vi "ProcessSpectralBands.vi"(8 "error in (no error)":errorcluster, 11 "tdms ref in":refnum<k34>) -> (0 "error out":errorcluster, 3 "tdms ref out":refnum<k34>)   [LabVIEW 2017, in "DataExplorerSupport.lvlib"]
uses:
  <vilib>/addons/InsightCM/Utilities/DataExplorerSupport/DataExplorerSupport.lvlib
  <vilib>/addons/InsightCM/Utilities/Tdms/Tdms.lvlib
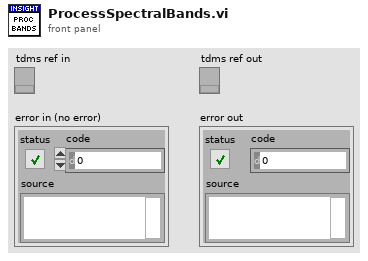
[diagram p1: front panel]
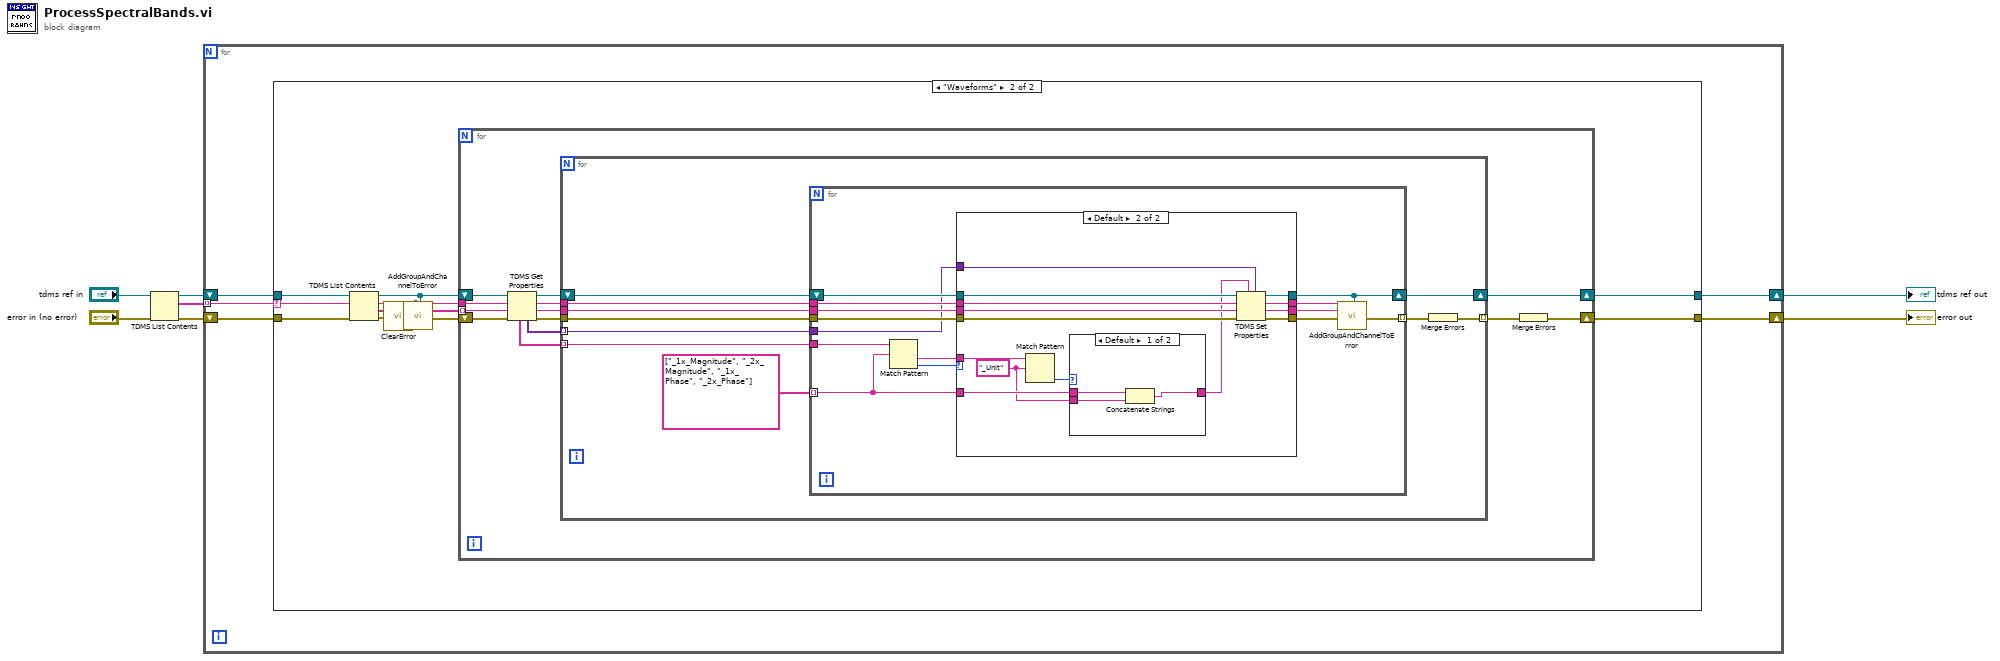
[diagram p0: block diagram]
diagram:
  n1 = TDMS List Contents(4:"error in (no error)", 7:"tdms ref in") -> (0:w2:errorcluster, 2:w1:string[], 3:w4:refnum<k34>)  [unwired: 1 in, 1 out]
  n2 = for {
    shift-right: [w11] -> w6
    shift-left: w4 -> [w10]
    shift-right: [w12] -> w7
    shift-left: w2 -> [w9]
    tunnel: w1 -> [w8] mode=indexing
    n3 = case shown="\"Waveforms\"" w8 {
      selector: w8 -> [_ w15]
      tunnel: [w13 w25] -> w12
      tunnel: [w14 w20] -> w11
      tunnel: w10 -> [w14 w17]
      tunnel: w9 -> [w13 w16]
      frame Default {
      }
      frame "Waveforms" {
        n4 = TDMS List Contents(4:w16, 6:w15, 7:w17) -> (0:w18:errorcluster, 1:w19:string[], 2:w23:string, 3:w24:refnum<k34>)
        n5 = call <vilib>:"ClearError.vi"("error in (no error)"=w18) -> ("error out"=w21:errorcluster)
        n6 = call <vilib>:"AddGroupAndChannelToError.vi"("error in (no error)"=w21, "group name in"=w23, "Refnum in"=w24) -> ("error out"=w22:errorcluster)  [unwired: 16 in]
        n7 = for {
          tunnel: w19 -> [w35] mode=indexing
          tunnel: w23 -> [w36]
          shift-right: [w27] -> w25
          shift-left: w22 -> [w38]
          shift-right: [w26] -> w20
          shift-left: w24 -> [w37]
          n8 = TDMS Get Properties(8:w38, 9:w35, 10:w36, 11:w37) -> (0:w30:errorcluster, 1:w31:string, 2:w32:string, 3:w33:refnum<k34>, 4:w29:variant[], 6:w34:string[])  [unwired: 2 in]
          n9 = for {
            tunnel: w34 -> [w48] mode=indexing
            tunnel: w32 -> [w45]
            tunnel: w31 -> [w46]
            tunnel: w30 -> [w47]
            tunnel: w29 -> [w43] mode=indexing
            tunnel: [w40] -> w28 mode=indexing
            shift-right: [w39] -> w26
            shift-left: w33 -> [w44]
            n10 = for {
              tunnel: w48 -> [w62]
              tunnel: w47 -> [w59]
              tunnel: w46 -> [w58]
              tunnel: w45 -> [w57]
              tunnel: w43 -> [w55]
              tunnel: string[] ["_1x_Magnitude", "_2x_Magnitude", "_1x_Phase", "_2x_Phase"] -> [w54] mode=indexing
              tunnel: [w50] -> w41 mode=indexing
              shift-right: [w49] -> w39
              shift-left: w44 -> [w56]
              n11 = Match Pattern(string=w62, regular expression=w54) -> (after substring=w60:string, offset past match=w61:i32)  [unwired: 1 in, 2 out]
              n12 = case shown="Default" w61 {
                tunnel: w60 -> [_ w80]
                tunnel: w59 -> [w63 w76]
                tunnel: w58 -> [w64 w77]
                tunnel: w57 -> [w65 w78]
                tunnel: w56 -> [w66 w79]
                tunnel: [w66 w68] -> w49
                tunnel: [w65 w69] -> w51
                tunnel: [w64 w70] -> w52
                tunnel: [w63 w71] -> w53
                tunnel: w54 -> [_ w73]
                tunnel: w55 -> [_ w75]
                frame -1 {
                }
                frame Default {
                  w67 = "_Unit" ("regular expression")
                  n13 = Match Pattern(string=w80, regular expression=w67) -> (offset past match=w74:i32)  [unwired: 1 in, 3 out]
                  n14 = case shown="Default" w74 {
                    tunnel: w73 -> [w83 w84]
                    tunnel: [w81 w84] -> w72
                    tunnel: w67 -> [w82 _]
                    frame Default {
                      n15 = Concatenate Strings(w83, w82) -> (w81:string)
                    }
                    frame -1 {
                    }
                  }
                  n16 = TDMS Set Properties(5:w75, 7:w72, 8:w76, 9:w77, 10:w78, 11:w79) -> (0:w71:errorcluster, 1:w70:string, 2:w69:string, 3:w68:refnum<k34>)
                }
              }
              n17 = call <vilib>:"AddGroupAndChannelToError.vi"("error in (no error)"=w53, "channel name in"=w52, "group name in"=w51, "Refnum in"=w49) -> ("error out"=w50:errorcluster)  [unwired: 15 in]
            }
            n18 = Merge Errors(w41) -> (w40:errorcluster)
          }
          n19 = Merge Errors(w28) -> (w27:errorcluster)
        }
      }
    }
  }
  "error out" <- w7
  "tdms ref out" <- w6
